vi "Normalize Type String.vi"(8 "Error In":errorcluster, 11 "Name":string) -> (0 "Error Out":errorcluster, 3 "normalized Name":string)   [LabVIEW 2011]
doc: "This VI normalizes the device type name. \"-\" is replaced by \" \" due to compatibility and the Version is deleted."
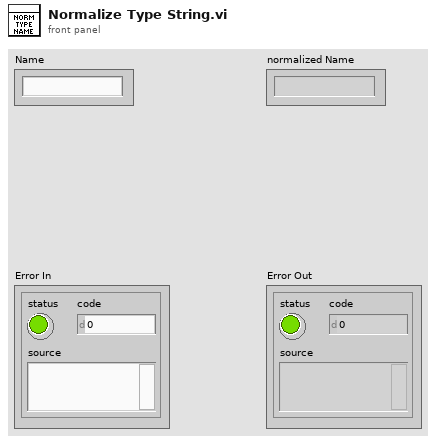
[diagram p1: front panel]
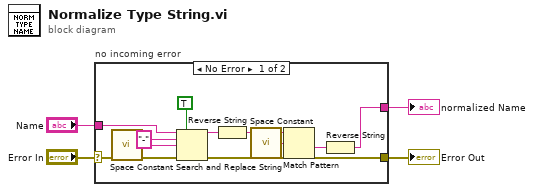
[diagram p0: block diagram]
diagram:
  n1 = case "no incoming error" shown="No Error" "Error In" {
    selector: "Error In" -> [w7 w17]
    tunnel: [w6 w17] -> w3
    tunnel: "Name" -> [w8 w16]
    tunnel: [w5 w16] -> w1
    frame No Error {
      n2 = call <vilib>:"Space Constant.vi"() -> ("String"=w9:string)
      n3 = Search and Replace String(replace all?=TRUE ("replace all? (F)"), input string=w8, search string="-", replace string=w9, error in=w7) -> (result string=w12:string, error out=w6:errorcluster)  [unwired: 3 in, 2 out]
      n4 = Reverse String(1:w12) -> (0:w15:string)
      n5 = call <vilib>:"Space Constant.vi"() -> ("String"=w14:string)
      n6 = Match Pattern(string=w15, regular expression=w14) -> (after substring=w13:string)  [unwired: 1 in, 3 out]
      n7 = Reverse String(1:w13) -> (0:w5:string)
    }
    frame Error {
    }
  }
  "Error Out" <- w3
  "normalized Name" <- w1
